vi "XY Graph Rebin Multiple Plots.vi"(8 "error in (no error)":errorcluster, 10 "Selected Plots":i32[](array[numeric]), 11 "Selected Plot Info":T1) -> (0 "error out":errorcluster, 1 "Rebinned Plot Message":string, 3 "Last Rebinned Plot":cluster{"t Array":dbl[], "IRF Array":dbl[]}, 4 "Single Plot?":bool)   [LabVIEW 2021, in "XY Graph Add-Ons.lvlib"]
uses:
  XY Graph Add-Ons.lvlib
  XY Graph Selected Plot Info.ctl
  XY Graph Refnum.ctl
  <vilib>/Utility/miscctls.llb/LVPoint32TypeDef.ctl
  Strings/Strings.lvlib
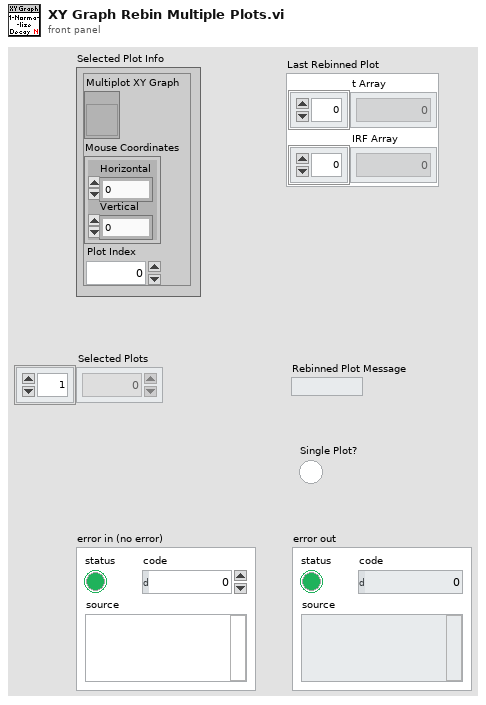
[diagram p1: front panel]
types:
  T1 = typedef "XY Graph Add-Ons.lvlib/XY Graph Selected Plot Info.ctl" = cluster{"Multiplot XY Graph":T2, "Mouse Coordinates":T3, "Plot Index":i32}
  T2 = typedef "XY Graph Add-Ons.lvlib/XY Graph Refnum.ctl" = refnum<vi>
  T3 = typedef "LVPoint32TypeDef.ctl" = cluster{"Horizontal":i32, "Vertical":i32}
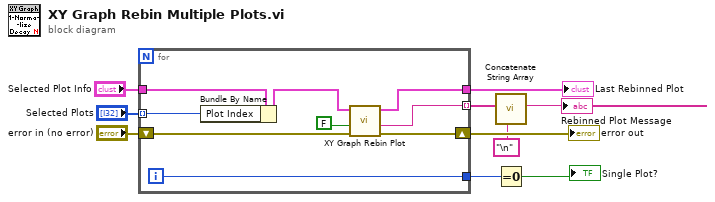
[diagram p0: block diagram]
diagram:
  n1 = for {
    tunnel: "Selected Plot Info" -> [w19]
    tunnel: [w11] -> w8 mode=indexing
    tunnel: [w13] -> w6
    shift-right: [w12] -> w7
    shift-left: "error in (no error)" -> [w16]
    tunnel: "Selected Plots" -> [w18] mode=indexing
    tunnel: [w17] -> w2
    i -> [w17]
    n2 = Bundle By Name(cluster=w19, "Plot Index"=w18) -> (w15:T1)
    n3 = call "XY Graph Rebin Plot.vi"("error in (no error)"=w16, "Replace Plot (T)?"=FALSE, "Selected Plot Info"=w15) -> ("Error Out"=w12:errorcluster, "Rebinned Plot Message"=w11:string, "Rebinned Plot"=w13:cluster{"t Array":dbl[], "IRF Array":dbl[]})  [unwired: 6 in]
  }
  "error out" <- w7
  "Last Rebinned Plot" <- w6
  n4 = call "Concatenate String Array.vi"("Separator (TAB)"="\n", "String Array"=w8) -> ("Formatted String"=→"Rebinned Plot Message":string)  [unwired: 9 in]
  n5 = Equal To 0?(x=w2) -> (x = 0?=→"Single Plot?":bool)
